vi "Path as Path.vi"   [LabVIEW 2020, in "G-Unicode.lvlib"]
uses:
  G-Unicode.lvlib
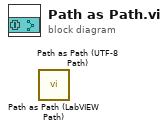
[diagram p0: block diagram]
diagram:
  n1 = call "Path as Path (LabVIEW Path).vi"() -> ()  [unwired: 11 in, 1 out]
  n2 = call "Path as Path (UTF-8 Path).vi"() -> ()  [unwired: 11 in, 1 out]
